vi "AddSubVI.vi"(5 "SubVI":refnum<class "SubVI.lvclass">, 6 "error in":errorcluster, 9 "PythonConverter_BD in":refnum<class "PyConvBD.lvclass">) -> (0 "error out":errorcluster, 3 "PythonConverter_BD out":refnum<class "PyConvBD.lvclass">)   [LabVIEW 2014, in "PyConvBD.lvclass"]
uses:
  PyConvBD.lvclass
  VI Interpreter/Classes/SubVI/SubVI.lvclass
  PyConvBD.lvclass/PyConvBD.ctl
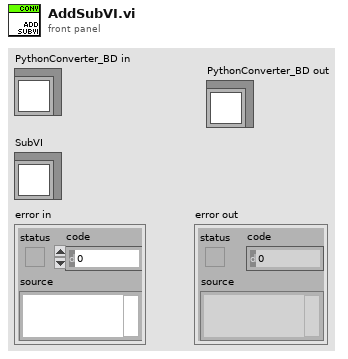
[diagram p1: front panel]
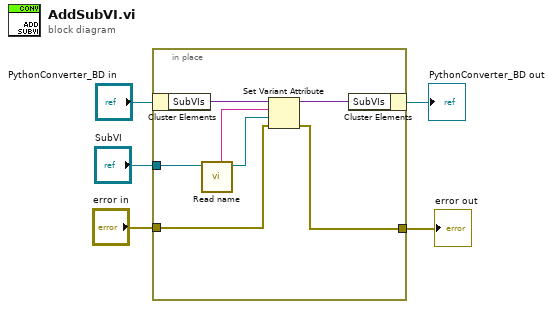
[diagram p0: block diagram]
diagram:
  n1 = in-place {
    in-place-border: "error in" -> [w11]
    in-place-border: [w10] -> w3
    in-place-border: "SubVI" -> [w8]
    n2 = in-place-cluster #1("PythonConverter_BD in") -> ("SubVIs"=w9:variant)
    n3 = call-dynamic "Read name.vi"("Node in"=w8) -> ("Node out"=w7:refnum<class "SubVI.lvclass">, "name"=w6:string)  [unwired: 7 in]
    n4 = Set Variant Attribute(Variant=w9, name=w6, value=w7, error in=w11) -> (Variant out=w12:variant, error out=w10:errorcluster)  [unwired: 1 out]
    n5 = in-place-cluster #1("SubVIs"=w12) -> (→"PythonConverter_BD out":refnum<class "PyConvBD.lvclass">)
  }
  "error out" <- w3
